vi "PC.vi"(11 "DataIn":T4) -> (3 "DataOut":T1)   [LabVIEW 2017]
doc: "SubVI criada para realizar a jogada do PC em caso de partida Player x PC"
uses:
  controls/DataIn.ctl
  controls/Tabuleiro.ctl
  controls/GameOption.ctl
  controls/DataOut.ctl
  controls/TabuleiroCoordenadas.ctl
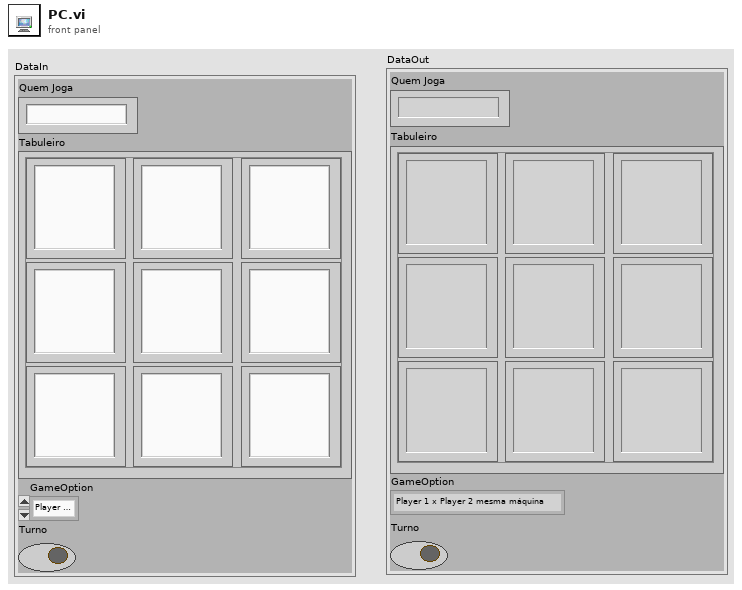
[diagram p1: front panel]
types:
  T1 = typedef "DataOut.ctl" = cluster{"Quem Joga":string, "Tabuleiro":T2, "GameOption":T3, "Turno":bool}
  T2 = typedef "Tabuleiro.ctl" = cluster{"(0,0)":string, "(1,0)":string, "(0,1)":string, "(1,1)":string, "(2,0)":string, "(1,2)":string, "(2,2)":string, "(0,2)":string, "(2,1) ":string}
  T3 = typedef "GameOption.ctl" = enum16{"Player 1 x Player 2 mesma máquina", "Player 1 x Player 2 pela rede", "Player 1 x Computador"}
  T4 = typedef "DataIn.ctl" = cluster{"Quem Joga":string, "Tabuleiro":T2, "GameOption":T3, "Turno":bool}
  T5 = typedef "TabuleiroCoordenadas.ctl" = enum16{"0,0", "0,1", "0,2", "1,0", "1,1", "1,2", "2,0", "2,1", "2,2"}
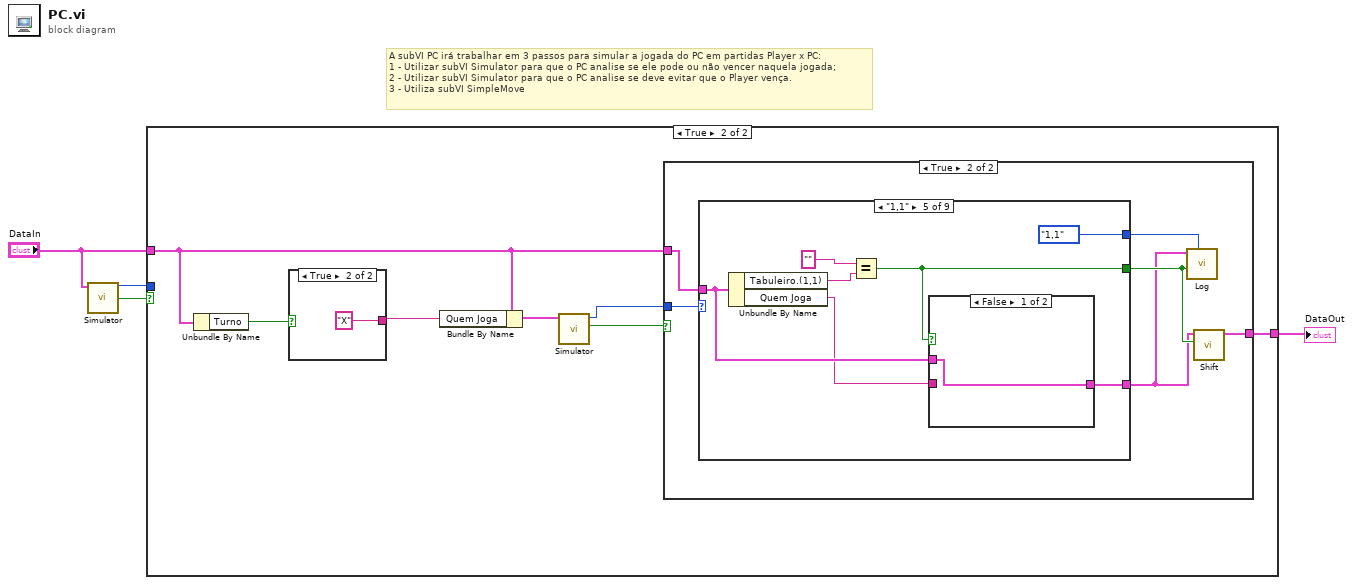
[diagram p0: block diagram]
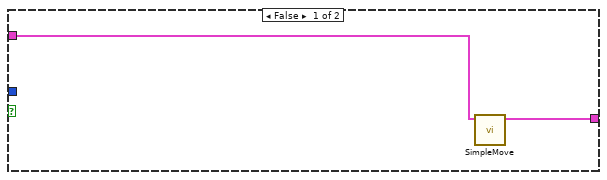
[diagram p3: hidden frame]
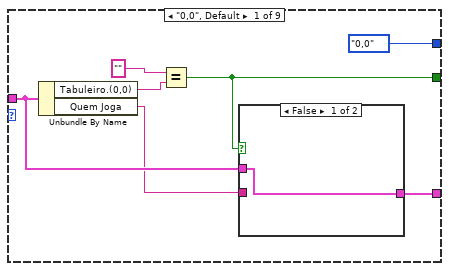
[diagram p4: hidden frame]
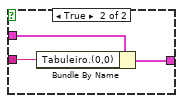
[diagram p5: hidden frame]
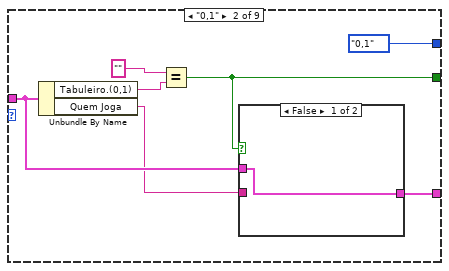
[diagram p6: hidden frame]
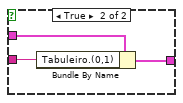
[diagram p7: hidden frame]
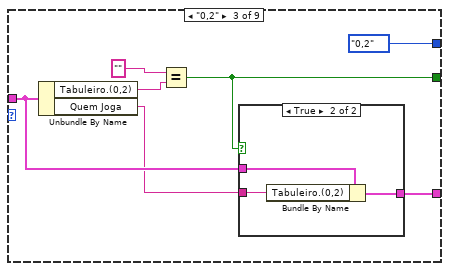
[diagram p8: hidden frame]
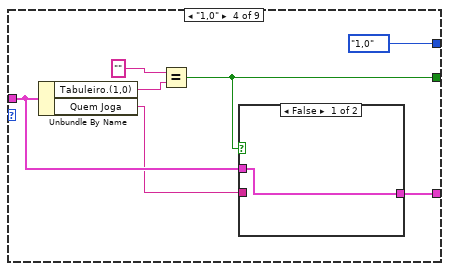
[diagram p10: hidden frame]
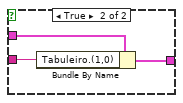
[diagram p11: hidden frame]
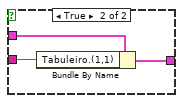
[diagram p12: hidden frame]
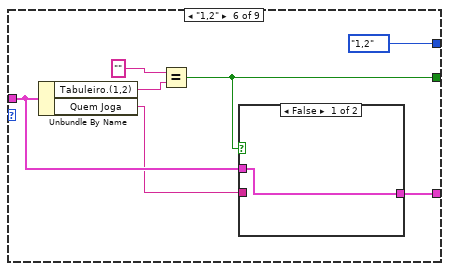
[diagram p13: hidden frame]
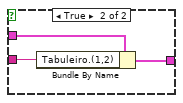
[diagram p14: hidden frame]
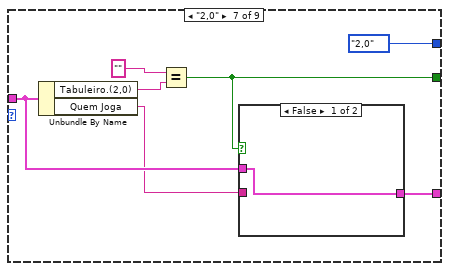
[diagram p15: hidden frame]
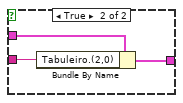
[diagram p16: hidden frame]
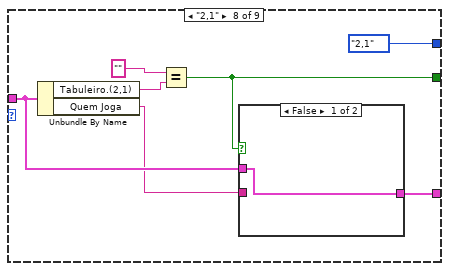
[diagram p17: hidden frame]
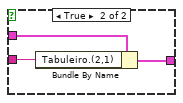
[diagram p18: hidden frame]
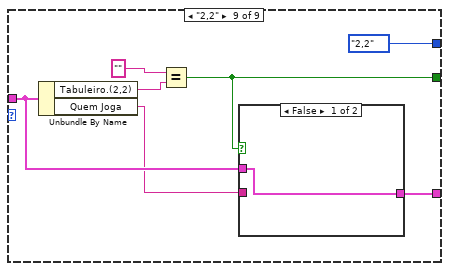
[diagram p19: hidden frame]
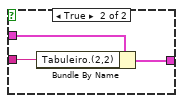
[diagram p20: hidden frame]
diagram:
  # "A subVI PC irá trabalhar em 3 passos para simular a jogada do PC em partidas Player x PC:\n1 - Utilizar subVI Simulator para que o PC analise se ele pode ou não vencer naquela jogada;\n2 - Utilizar subVI Simulator para que o PC analise se deve evitar que o Player vença.\n3 - Utiliza subVI SimpleMove"
  n1 = call "Simulator.vi"("DataIn"="DataIn") -> ("true = ganhou"=w3:bool, "Enum"=w2:T5)  [unwired: 9 in]
  n2 = case shown="True" w3 {
    tunnel: "DataIn" -> [w5 w7]
    tunnel: w2 -> [_ _]
    tunnel: [w5 w6] -> w1
    frame False {
    }
    frame True {
      n3 = Unbundle By Name(w7) -> ("Turno"=w12:bool)
      n4 = case shown="True" w12 {
        tunnel: ["O" "X"] -> w11
        frame False {
        }
        frame True {
        }
      }
      n5 = Bundle By Name(cluster=w7, "Quem Joga"=w11) -> (w10:T4)
      n6 = call "Simulator.vi"("DataIn"=w10) -> ("true = ganhou"=w9:bool, "Enum"=w8:T5)  [unwired: 9 in]
      n7 = case shown="True" w9 {
        tunnel: w8 -> [_ w20]
        tunnel: w7 -> [w13 w19]
        tunnel: [w14 w15] -> w6
        frame False {
          n8 = call "SimpleMove.vi"("DataIn"=w13) -> ("DataOut"=w14:T1)  [unwired: 10 in]
        }
        frame True {
          n9 = case shown="\"1,1\"" w20 {
            tunnel: w19 -> [w24 w35 w46 w57 w68 w79 w90 w101 w112]
            tunnel: [w25 w36 w47 w58 w69 w80 w91 w102 w113] -> w17
            tunnel: [w22 w33 w44 w55 w66 w77 w88 w99 w110] -> w16
            tunnel: [TabuleiroCoordenadas."0,0" ("Enum") TabuleiroCoordenadas."0,1" ("Enum") TabuleiroCoordenadas."0,2" ("Enum") TabuleiroCoordenadas."1,0" ("Enum") TabuleiroCoordenadas."1,1" ("Enum") TabuleiroCoordenadas."1,2" ("Enum") TabuleiroCoordenadas."2,0" ("Enum") TabuleiroCoordenadas."2,1" ("Enum") TabuleiroCoordenadas."2,2" ("Enum")] -> w18
            frame "0,0", Default {
              n10 = Unbundle By Name(w24) -> ("Tabuleiro.(0,0)"=w27:string, "Quem Joga"=w23:string)
              n11 = Equal?(x="", y=w27) -> (x = y?=w25:bool)
              n12 = case shown="False" w25 {
                tunnel: w24 -> [w28 w31]
                tunnel: w23 -> [_ w30]
                tunnel: [w28 w29] -> w22
                frame False {
                }
                frame True {
                  n13 = Bundle By Name(cluster=w31, "Tabuleiro.(0,0)"=w30) -> (w29:T4)
                }
              }
            }
            frame "0,1" {
              n14 = Unbundle By Name(w35) -> ("Tabuleiro.(0,1)"=w38:string, "Quem Joga"=w34:string)
              n15 = Equal?(x="", y=w38) -> (x = y?=w36:bool)
              n16 = case shown="False" w36 {
                tunnel: w35 -> [w39 w42]
                tunnel: w34 -> [_ w41]
                tunnel: [w39 w40] -> w33
                frame False {
                }
                frame True {
                  n17 = Bundle By Name(cluster=w42, "Tabuleiro.(0,1)"=w41) -> (w40:T4)
                }
              }
            }
            frame "0,2" {
              n18 = Unbundle By Name(w46) -> ("Tabuleiro.(0,2)"=w49:string, "Quem Joga"=w45:string)
              n19 = Equal?(x="", y=w49) -> (x = y?=w47:bool)
              n20 = case shown="True" w47 {
                tunnel: w46 -> [w50 w53]
                tunnel: w45 -> [_ w52]
                tunnel: [w50 w51] -> w44
                frame False {
                }
                frame True {
                  n21 = Bundle By Name(cluster=w53, "Tabuleiro.(0,2)"=w52) -> (w51:T4)
                }
              }
            }
            frame "1,0" {
              n22 = Unbundle By Name(w57) -> ("Tabuleiro.(1,0)"=w60:string, "Quem Joga"=w56:string)
              n23 = Equal?(x="", y=w60) -> (x = y?=w58:bool)
              n24 = case shown="False" w58 {
                tunnel: w57 -> [w61 w64]
                tunnel: w56 -> [_ w63]
                tunnel: [w61 w62] -> w55
                frame False {
                }
                frame True {
                  n25 = Bundle By Name(cluster=w64, "Tabuleiro.(1,0)"=w63) -> (w62:T4)
                }
              }
            }
            frame "1,1" {
              n26 = Unbundle By Name(w68) -> ("Tabuleiro.(1,1)"=w71:string, "Quem Joga"=w67:string)
              n27 = Equal?(x="", y=w71) -> (x = y?=w69:bool)
              n28 = case shown="False" w69 {
                tunnel: w68 -> [w72 w75]
                tunnel: w67 -> [_ w74]
                tunnel: [w72 w73] -> w66
                frame False {
                }
                frame True {
                  n29 = Bundle By Name(cluster=w75, "Tabuleiro.(1,1)"=w74) -> (w73:T4)
                }
              }
            }
            frame "1,2" {
              n30 = Unbundle By Name(w79) -> ("Tabuleiro.(1,2)"=w82:string, "Quem Joga"=w78:string)
              n31 = Equal?(x="", y=w82) -> (x = y?=w80:bool)
              n32 = case shown="False" w80 {
                tunnel: w79 -> [w83 w86]
                tunnel: w78 -> [_ w85]
                tunnel: [w83 w84] -> w77
                frame False {
                }
                frame True {
                  n33 = Bundle By Name(cluster=w86, "Tabuleiro.(1,2)"=w85) -> (w84:T4)
                }
              }
            }
            frame "2,0" {
              n34 = Unbundle By Name(w90) -> ("Tabuleiro.(2,0)"=w93:string, "Quem Joga"=w89:string)
              n35 = Equal?(x="", y=w93) -> (x = y?=w91:bool)
              n36 = case shown="False" w91 {
                tunnel: w90 -> [w94 w97]
                tunnel: w89 -> [_ w96]
                tunnel: [w94 w95] -> w88
                frame False {
                }
                frame True {
                  n37 = Bundle By Name(cluster=w97, "Tabuleiro.(2,0)"=w96) -> (w95:T4)
                }
              }
            }
            frame "2,1" {
              n38 = Unbundle By Name(w101) -> ("Tabuleiro.(2,1)"=w104:string, "Quem Joga"=w100:string)
              n39 = Equal?(x="", y=w104) -> (x = y?=w102:bool)
              n40 = case shown="False" w102 {
                tunnel: w101 -> [w105 w108]
                tunnel: w100 -> [_ w107]
                tunnel: [w105 w106] -> w99
                frame False {
                }
                frame True {
                  n41 = Bundle By Name(cluster=w108, "Tabuleiro.(2,1)"=w107) -> (w106:T4)
                }
              }
            }
            frame "2,2" {
              n42 = Unbundle By Name(w112) -> ("Tabuleiro.(2,2)"=w115:string, "Quem Joga"=w111:string)
              n43 = Equal?(x="", y=w115) -> (x = y?=w113:bool)
              n44 = case shown="False" w113 {
                tunnel: w112 -> [w116 w119]
                tunnel: w111 -> [_ w118]
                tunnel: [w116 w117] -> w110
                frame False {
                }
                frame True {
                  n45 = Bundle By Name(cluster=w119, "Tabuleiro.(2,2)"=w118) -> (w117:T4)
                }
              }
            }
          }
          n46 = call "Log.vi"("Enum Coordenadas"=w18, "Confirmação"=w17, "DataIn"=w16) -> ()  [unwired: 7 in, 2 out]
          n47 = call "Shift.vi"("Confirmação"=w17, "DataIn"=w16) -> ("DataOut"=w15:T1)  [unwired: 7 in, 2 out]
        }
      }
    }
  }
  "DataOut" <- w1
